vi "Encode string.vi"(11 "string":string) -> (3 "encoded string":string)   [LabVIEW 2020]
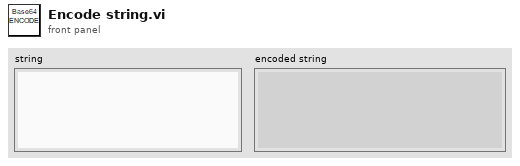
[diagram p1: front panel]
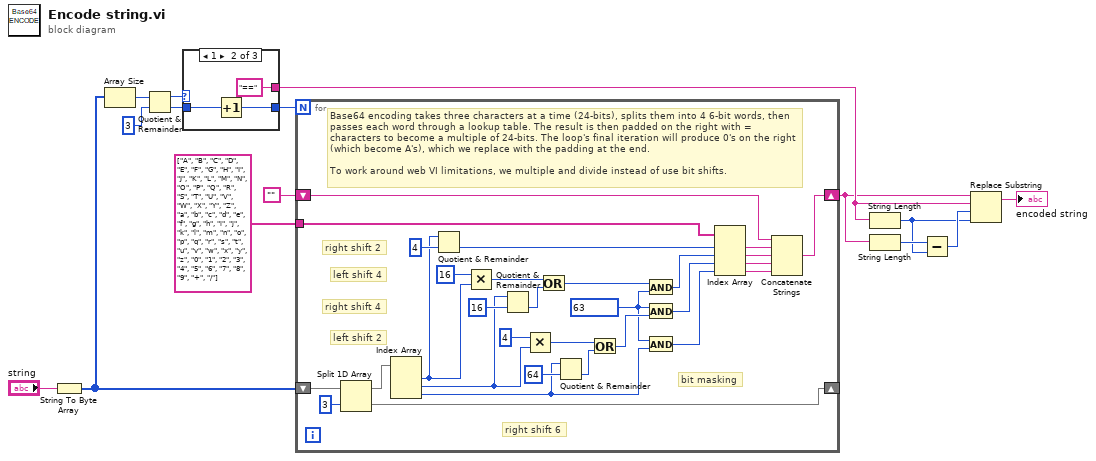
[diagram p0: block diagram]
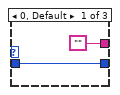
[diagram p2: hidden frame]
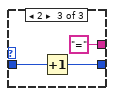
[diagram p3: hidden frame]
diagram:
  n1 = String To Byte Array(string="string") -> (unsigned byte array=w2:u8[])
  n2 = Array Size(array=w2) -> (size(s)=w14:i32)
  n3 = Quotient & Remainder(x=w14, y=3) -> (x-y*floor(x/y)=w9:i32, floor(x/y)=w12:i32)
  n4 = case shown="1" w9 {
    tunnel: w12 -> [w17 w20 w23]
    tunnel: [w17 w19 w22] -> w1
    tunnel: ["" "==" "="] -> w7
    frame 0, Default {
    }
    frame 1 {
      n5 = Increment(x=w20) -> (x+1=w19:i32)
    }
    frame 2 {
      n6 = Increment(x=w23) -> (x+1=w22:i32)
    }
  }
  n7 = for {
    N: w1 -> [_]
    tunnel: string[] ["A", "B", "C", "D", "E", "F", "G", "H", "I", "J", "K", "L", "M", "N", "O", "P", "Q", "R", "S", "T", "U", "V", "W", "X", "Y", "Z", "a", "b", "c", "d", "e", "f", "g", "h", "i", "j", "k", "l", "m", "n", "o", "p", "q", "r", "s", "t", "u", "v", "w", "x", "y", "z", "0", "1", "2", "3", "4", "5", "6", "7", "8", "9", "+", "/"] -> [w47]
    shift-right: [w32] -> w5
    shift-left: "" -> [w31]
    shift-right: [w29] -> _
    shift-left: w2 -> [w30]
    w37 = u8 63 ("y")
    # "bit masking"
    # "right shift 6"
    # "left shift 2"
    # "right shift 4"
    # "left shift 4"
    # "right shift 2"
    # "Base64 encoding takes three characters at a time (24-bits), splits them into 4 6-bit words, then passes each word through a lookup table. The result is then padded on the right with = characters to become a multiple of 24-bits. The loop's final iteration will produce 0's on the right (which become A's), which we replace with the padding at the end.\n\nTo work around web VI limitations, we multiple and divide instead of use bit shifts."
    n8 = Split 1D Array(array=w30, index=3) -> (first subarray=w52:u8[], second subarray=w29:u8[])
    n9 = Index Array(array=w52) -> (element #1=w25:u8, element #2=w50:u8, element #3=w39:u8)  [unwired: 3 in]
    n10 = Quotient & Remainder(x=w25, y=u8 4) -> (floor(x/y)=w28:u8)  [unwired: 1 out]
    n11 = Multiply(x=u8 16 ("y"), y=w25) -> (x*y=w24:u8)
    n12 = Quotient & Remainder(x=w50, y=u8 16) -> (floor(x/y)=w46:u8)  [unwired: 1 out]
    n13 = Multiply(x=u8 4 ("y"), y=w50) -> (x*y=w45:u8)
    n14 = Or(x=w24, y=w46) -> (x .or. y?=w43:u8)
    n15 = Quotient & Remainder(x=w39, y=u8 64) -> (floor(x/y)=w44:u8)  [unwired: 1 out]
    n16 = Or(x=w45, y=w44) -> (x .or. y?=w41:u8)
    n17 = And(x=w43, y=w37) -> (x .and. y?=w42:u8)
    n18 = And(x=w37, y=w41) -> (x .and. y?=w40:u8)
    n19 = And(x=w37, y=w39) -> (x .and. y?=w38:u8)
    n20 = Index Array(array=w47, index #1=w28, index #2=w42, index #3=w40, index #4=w38) -> (element #1=w36:string, element #2=w35:string, element #3=w34:string, element #4=w33:string)
    n21 = Concatenate Strings(w31, w36, w35, w34, w33) -> (w32:string)
  }
  n22 = String Length(string=w7) -> (length=w6:i32)
  n23 = String Length(string=w5) -> (length=w11:i32)
  n24 = Subtract(x=w11, y=w6) -> (x-y=w10:i32)
  n25 = Replace Substring(2:w6, 3:w10, 4:w7, 5:w5) -> (1:→"encoded string":string)  [unwired: 1 out]
